vi "CSVsavevi.vi"(8 "error in (no error)":errorcluster, 10 "Input array":dbl[](array[numeric]), 11 "file path (dialog if empty)":path) -> (0 "error out":errorcluster)   [LabVIEW 2022 SP3]
uses:
  <vilib>/Utility/file.llb/Write Delimited Spreadsheet (string).vi
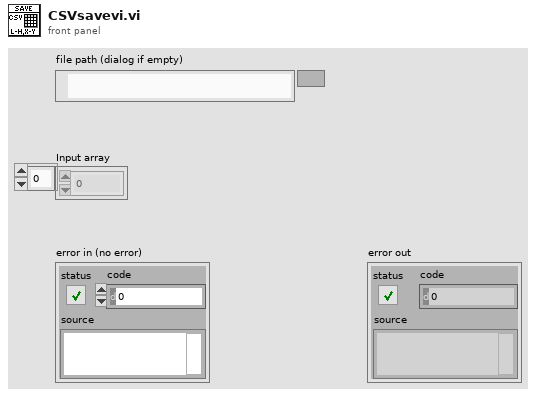
[diagram p1: front panel]
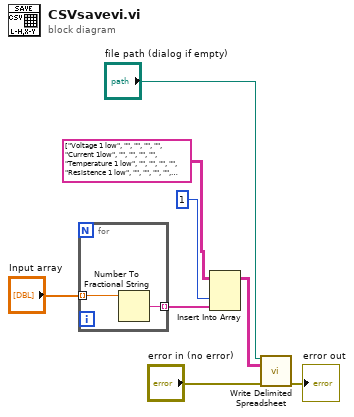
[diagram p0: block diagram]
diagram:
  n1 = for {
    tunnel: "Input array" -> [w10] mode=indexing
    tunnel: [w9] -> w4 mode=indexing
    n2 = Number To Fractional String(number=w10) -> (F-format string=w9:string)  [unwired: 3 in]
  }
  n3 = Insert Into Array(array=string[][] [["Voltage 1 low", "", "", "", ""], ["Current 1low", "", "", "", ""], ["Temperature 1 low", "", "", "", ""], ["Resistence 1 low", "", "", "", ""], ["Voltage 1 High", "", "", "", ""], ["Current 1 High", "", "", "", ""], ["Temperature 1 High", "", "", "", ""], ["Resistence 1 High", "", "", "", ""], ["Xaxis", "", "", "", ""], ["Yaxis", "", "", "", ""], ["Voltage 2 low", "", "", "", ""], ["Current 2 low", "", "", "", ""], ["Temperature 2 low", "", "", "", ""], ["Resistence 2 low", "", "", "", ""], ["Voltage 2 High", "", "", "", ""], ["Current 2 High", "", "", "", ""], ["Temperature 2 High", "", "", "", ""], ["Resistence 2 High", "", "", "", ""]], index (col)=1 ("disabled index (col)"), new element=w4) -> (w6:string[][])  [unwired: 1 in]
  n4 = call-poly <vilib>:"Write Delimited Spreadsheet.vi"("file path (dialog if empty)"="file path (dialog if empty)", "2D data"=w6, "error in (no error)"="error in (no error)") -> ("error out"=→"error out":errorcluster)  [unwired: 11 in, 1 out]
